vi "controller.vi"(0 "position":dbl, 1 "pos ref":dbl, 3 "velocity":dbl, 4 "vel ref":dbl, 7 "b_":dbl, 9 "k_":dbl) -> (15 "duty out":dbl, 17 "K1_c":dbl, 18 "K2_c":dbl)   [LabVIEW 2019]
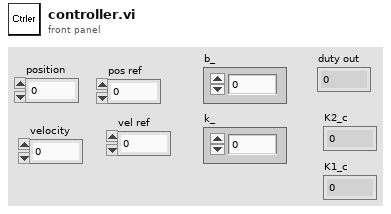
[diagram p1: front panel]
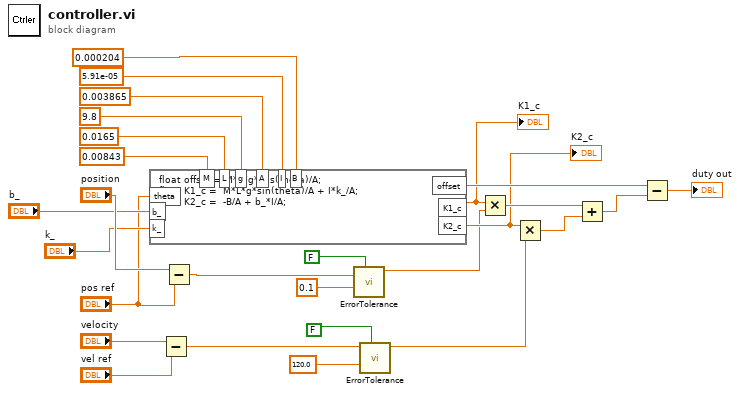
[diagram p0: block diagram]
diagram:
  n1 = formula code="float offset = M*L*g*cos(theta)/A;\nfloat K1_c =  M*L*g*sin(theta)/A + I*k_/A;\nfloat K2_c =  -B/A + b_*I/A;"("M"=0.00843 ("input variable"), "L"=0.0165 ("input variable"), "g"=9.8 ("input variable"), "theta"="pos ref", "A"=0.003865 ("input variable"), "b_"="b_", "k_"="k_", "I"=5.91e-05 ("input variable"), "B"=0.000204 ("input variable")) -> ("offset"=w25:dbl, "K1_c"=w13:dbl, "K2_c"=w11:dbl)
  "K1_c" <- w13
  "K2_c" <- w11
  n2 = Subtract(x="velocity", y="vel ref") -> (x-y=w3:dbl)
  n3 = Subtract(x="position", y="pos ref") -> (x-y=w9:dbl)
  n4 = call "ErrorTolerance.vi"("Enable"=FALSE, "error tol"=0.1, "input"=w9) -> ("output"=w10:dbl)  [unwired: 8 in]
  n5 = call "ErrorTolerance.vi"("Enable"=FALSE, "error tol"=120.0, "input"=w3) -> ("output"=w2:dbl)  [unwired: 8 in]
  n6 = Multiply(x=w13, y=w10) -> (x*y=w15:dbl)
  n7 = Multiply(x=w11, y=w2) -> (x*y=w14:dbl)
  n8 = Add(x=w15, y=w14) -> (x+y=w27:dbl)
  n9 = Subtract(x=w25, y=w27) -> (x-y=→"duty out":dbl)
